vi "update_mode.vi"(7 "references":T2, 8 "error in (no error)":errorcluster, 11 "mode":T1) -> (0 "error out":errorcluster)   [LabVIEW 2015, in "repub-dvr_nre.lvlib"]
uses:
  repub-dvr_nre.lvlib
  _controls/references.ctl
  private/_controls/input.ctl
  private/_controls/input_command.ctl
  private/_controls/output.ctl
  private/_controls/data.ctl
  _controls/configuration.ctl
  lv-recipe-machine/private/_controls/recipe_data.ctl
  lv-recipe-machine/public/_controls/mode.ctl
  lv-recipe-machine/public/_controls/manual_state.ctl
  lv-recipe-machine/public/_controls/automatic_state.ctl
  <userlib>/antonio-alexander/lv-waitgroup/public/_controls/api_waitgroup.ctl
  lv-recipe-machine/public/_controls/transition.ctl
  _controls/change.ctl
  _controls/status.ctl
  lv-recipe-machine/lv-recipe-machine.lvlib
  <userlib>/antonio-alexander/lv-waitgroup/lv-waitgroup.lvlib
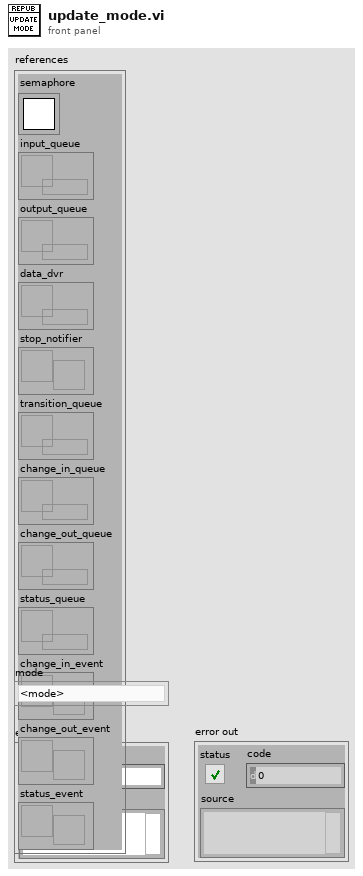
[diagram p1: front panel]
types:
  T1 = typedef "lv-recipe-machine.lvlib/mode.ctl" = enum16{"<mode>", "manual", "automatic", "<null>"}
  T2 = typedef "repub-dvr_nre.lvlib/references.ctl" = cluster{"semaphore":T3, "input_queue":refnum<queue>, "output_queue":refnum<queue>, "data_dvr":refnum<data-value>, "stop_notifier":refnum<notifier>, "transition_queue":refnum<queue>, "change_in_queue":refnum<queue>, "change_out_queue":refnum<queue>, "status_queue":refnum<queue>, "change_in_event":refnum<user-event>, "change_out_event":refnum<user-event>, "status_event":refnum<user-event>}
  T3 = typedef "Semaphore RefNum" = refnum<k1>
  T4 = typedef "lv-recipe-machine.lvlib/manual_state.ctl" = enum16{"<manual_state>", "failed", "action", "running", "idle", "<null>"}
  T5 = typedef "repub-dvr_nre.lvlib/data.ctl" = cluster{"configuration":T6, "working":cluster{"recipe_data":T7, "api_waitgroup":T9}}
  T6 = typedef "repub-dvr_nre.lvlib/configuration.ctl" = cluster{dbl}
  T7 = typedef "lv-recipe-machine.lvlib/recipe_data.ctl" = cluster{"mode":T1, "manual_state":T4, "automatic_state":T8, "step":string, "automatic_recipe":variant, "manual_actions":variant}
  T8 = typedef "lv-recipe-machine.lvlib/automatic_state.ctl" = enum16{"<automatic_state>", "failed", "idle", "running", "paused", "transition", "stopped", "<null>"}
  T9 = typedef "lv-waitgroup.lvlib/api_waitgroup.ctl" = cluster{"waitgroups":refnum<data-value>, "waitgroup":string}
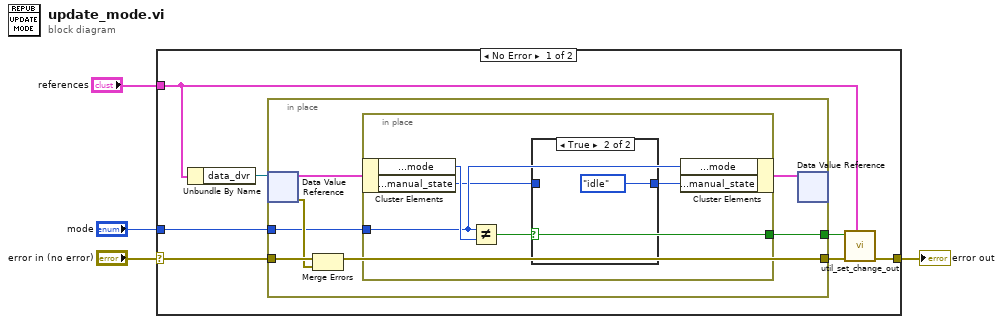
[diagram p0: block diagram]
diagram:
  n1 = case shown="No Error" "error in (no error)" {
    selector: "error in (no error)" -> [w10 w26]
    tunnel: [w5 w26] -> w3
    tunnel: "references" -> [w6 _]
    tunnel: "mode" -> [w9 _]
    frame No Error {
      n2 = Unbundle By Name(w6) -> ("data_dvr"=w11:refnum<data-value>)
      n3 = in-place {
        in-place-border: [w16] -> w8
        in-place-border: w10 -> [w18]
        in-place-border: w9 -> [w13]
        in-place-border: [w12] -> w7
        n4 = in-place-dvr #1(w11) -> (w15:T5, w17:errorcluster)
        n5 = Merge Errors(w18, w17) -> (w16:errorcluster)
        n6 = in-place {
          in-place-border: w13 -> [w22]
          in-place-border: [w21] -> w12
          n7 = in-place-cluster #2(w15) -> ("working.recipe_data.mode"=w23:T1, "working.recipe_data.manual_state"=w20:T4)
          n8 = Not Equal?(x=w22, y=w23) -> (x != y?=w21:bool)
          n9 = case shown="True" w21 {
            tunnel: w20 -> [w24 _]
            tunnel: [w24 manual_state."idle" ("manual_state")] -> w19
            frame False {
            }
            frame True {
            }
          }
          n10 = in-place-cluster #2("working.recipe_data.mode"=w22, "working.recipe_data.manual_state"=w19) -> (w14:T5)
        }
        n11 = in-place-dvr #1(w14) -> ()  [unwired: 2 out]
      }
      n12 = call "util_set_change_out.vi"("references"=w6, "error in (no error)"=w8, "change"=w7) -> ("error out"=w5:errorcluster)  [unwired: 8 in]
    }
    frame Error {
    }
  }
  "error out" <- w3
